vi "DTACQ - Verify AWG Length.vi"(8 "error in":errorcluster, 10 "Number of Samples Uploaded":i32, 11 "Address":string) -> (0 "error out":errorcluster, 2 "Timeout":bool)   [LabVIEW 2017, in "Communications Library.lvlib"]
doc: "Tests the reported length of the arbitrary waveform.\n \nThe VI exits, when either;\nthe length of the arbitrary waveform is equal to the expected length\nor\nthe timeout expires"
uses:
  Communications Library.lvlib
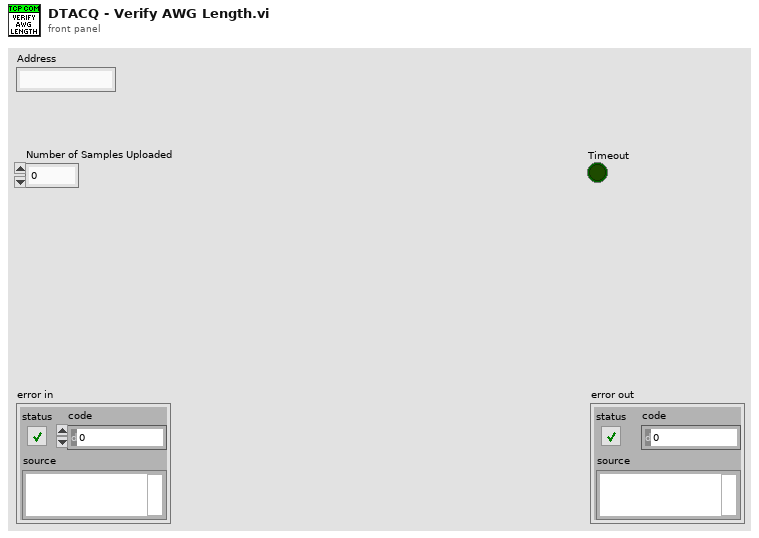
[diagram p1: front panel]
types:
  T1 = typedef "Communications Library.lvlib/DTACQ Module Configuration--Cluster.ctl" = cluster{"Name":string, "Position":string, "Module Type":T2, "Control Port":i32, "Timeout (ms)":i32, "Channels":i32}
  T2 = typedef "Communications Library.lvlib/DTACQ Device Type--Enum.ctl" = enum16{"Carrier", "Analog In Module", "Analog Out Module", "Generic Module"}
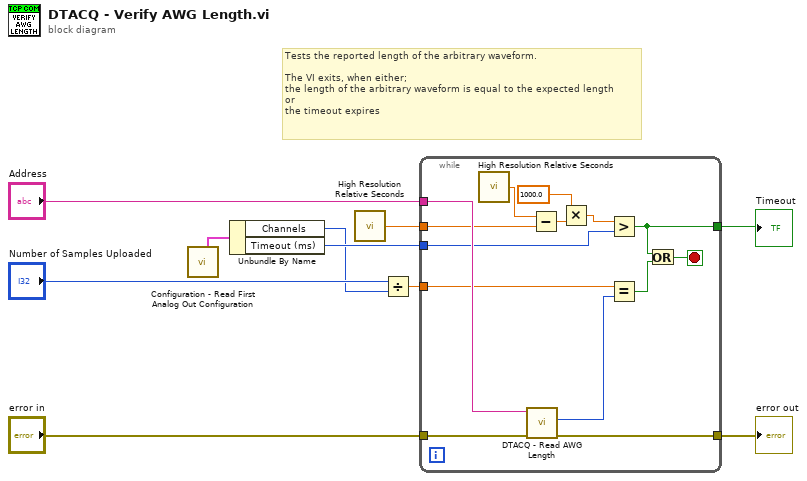
[diagram p0: block diagram]
diagram:
  # "Tests the reported length of the arbitrary waveform.\n \nThe VI exits, when either;\nthe length of the arbitrary waveform is equal to the expected length\nor\nthe timeout expires"
  n1 = call "Configuration - Read First Analog Out Configuration.vi"() -> ("AO - Module Configuration"=w4:T1)  [unwired: 7 in, 4 out]
  n2 = Unbundle By Name(w4) -> ("Channels"=w5:i32, "Timeout (ms)"=w9:i32)
  n3 = call <vilib>:"High Resolution Relative Seconds.vi"() -> ("relative seconds"=w8:dbl)
  n4 = Divide(x="Number of Samples Uploaded", y=w5) -> (x/y=w7:dbl)
  n5 = while {
    tunnel: "error in" -> [w24]
    tunnel: "Address" -> [w23]
    tunnel: w7 -> [w22]
    tunnel: w8 -> [w20]
    tunnel: w9 -> [w18]
    tunnel: [w15] -> w10
    tunnel: [w14] -> w1
    stop <- w17 stop-if-true
    n6 = call <vilib>:"High Resolution Relative Seconds.vi"() -> ("relative seconds"=w19:dbl)
    n7 = call "DTACQ - Read AWG Length.vi"("error in"=w24, "Address"=w23) -> ("error out"=w15:errorcluster, "AWG Length"=w21:i32)  [unwired: 8 in]
    n8 = Subtract(x=w19, y=w20) -> (x-y=w13:dbl)
    n9 = Multiply(x=1000.0, y=w13) -> (x*y=w11:dbl)
    n10 = Greater?(x=w11, y=w18) -> (0:w14:bool)
    n11 = Equal?(x=w22, y=w21) -> (x = y?=w16:bool)
    n12 = Or(x=w14, y=w16) -> (x .or. y?=w17:bool)
  }
  "error out" <- w10
  "Timeout" <- w1
